vi "SubName.vi"(8 "error in (no error)":errorcluster, 11 ".NET Refnum in":refnum<k24>) -> (0 "error out":errorcluster, 2 "SubjectName":string, 3 ".NET Refnum out":refnum<k24>)   [LabVIEW 2024]
uses:
  C:/Users/ROAR/Documents/Rob Motor Assessment stuff/Labview/RobUST_3D_with_Unity_Control_PXI_Low_Level_Only_Streamlined/Vicon_files/ViconDataStreamSDK_DotNET.dll
  Vicon_files/ViconDataStreamSDK_DotNET.dll
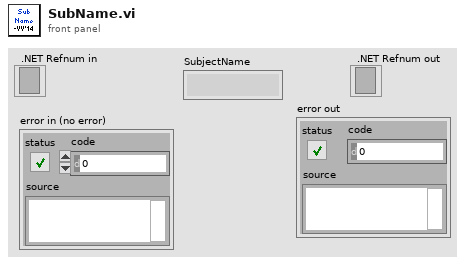
[diagram p1: front panel]
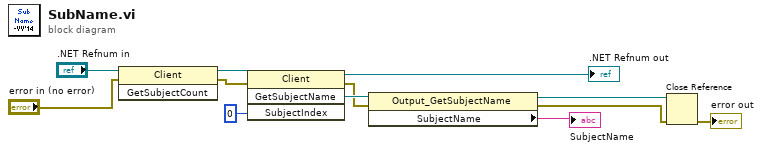
[diagram p0: block diagram]
diagram:
  n1 = invoke class="Client" method="GetSubjectCount"(reference=".NET Refnum in", error in="error in (no error)") -> (reference out=w7:refnum<k24>, error out=w5:errorcluster)  [unwired: 1 in, 1 out]
  n2 = invoke class="Client" method="GetSubjectName"(reference=w7, error in=w5, "SubjectIndex"=u32 0) -> (reference out=→".NET Refnum out":refnum<k24>, error out=w4:errorcluster, "GetSubjectName"=w8:refnum<k24>)  [unwired: 1 in, 1 out]
  n3 = property class="Output_GetSubjectName"(reference=w8, error in=w4) -> (reference out=w3:refnum<k24>, error out=w2:errorcluster, "SubjectName"=→"SubjectName":string)
  n4 = Close Reference(reference=w3, error in (no error)=w2) -> (error out=→"error out":errorcluster)
